vi "04 Loops.vi"() -> ()   [LabVIEW 2019]
uses:
  _Subs/OpenDiagram/Open_XControl.xctl
panel:
  in  "OpenDiag":refnum<vi>(xcontrol)
  out "Waveform Chart 3":i32[][](graph)
  out "Waveform Chart 2":i32(graph)
  out "Waveform Chart":i32(graph)
  # "04 Loops\nThis code compares while and for loops\n\nInstructions:\n1. Hit the Run arrow and see the plots change\n2. Look at the block diagram in Highlight Execution mode to see how data is fed to each chart"
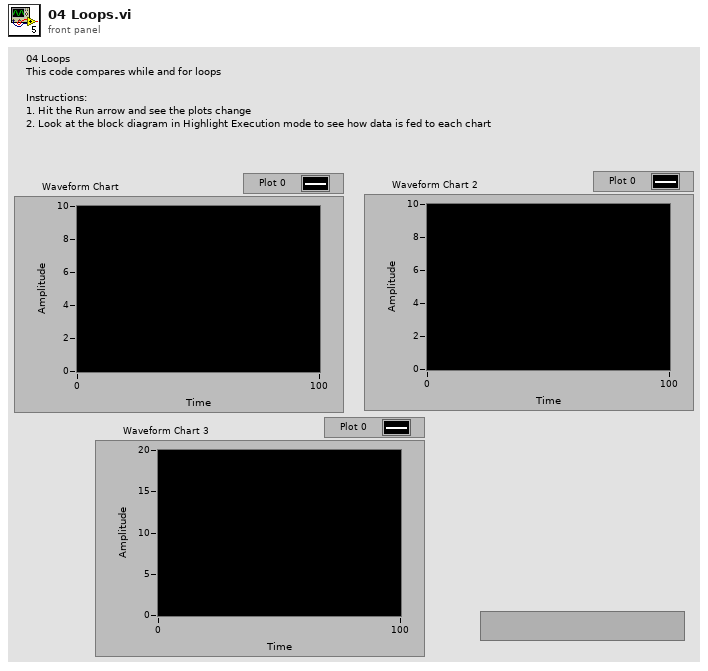
[diagram p1: front panel]
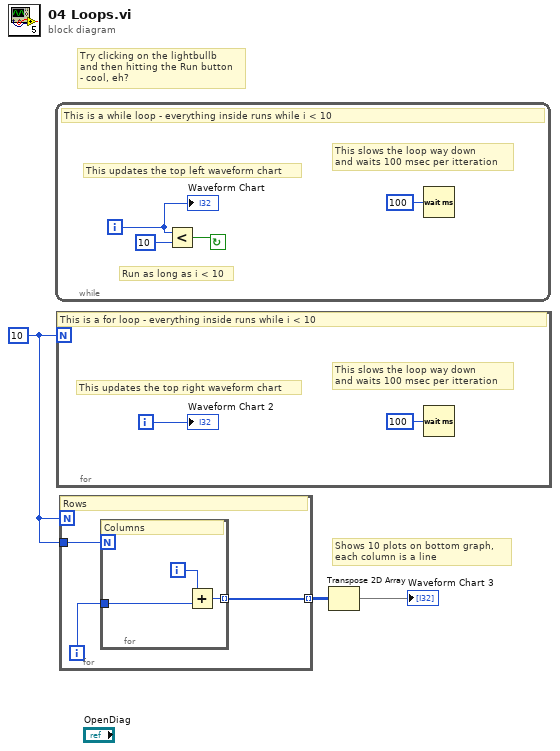
[diagram p0: block diagram]
diagram:
  w2 = 10
  # "Shows 10 plots on bottom graph,\neach column is a line"
  # "Try clicking on the lightbullb\nand then hitting the Run button\n- cool, eh?"
  n1 = while {
    i -> [w6]
    stop <- w4 continue-if-true
    # "Run as long as i < 10"
    # "This slows the loop way down \nand waits 100 msec per itteration"
    # "This updates the top left waveform chart"
    # "This is a while loop - everything inside runs while i < 10"
    n2 = Less?(x=w6, y=10) -> (x < y?=w4:bool)
    n3 = Wait (ms)(milliseconds to wait=u32 100) -> ()  [unwired: 1 out]
    "Waveform Chart" <- w6
  }
  n4 = for {
    N: w2 -> [_]
    i -> [w8]
    # "This slows the loop way down \nand waits 100 msec per itteration"
    # "This updates the top right waveform chart"
    # "This is a for loop - everything inside runs while i < 10"
    n5 = Wait (ms)(milliseconds to wait=u32 100) -> ()  [unwired: 1 out]
    "Waveform Chart 2" <- w8
  }
  n6 = for {
    N: w2 -> [_]
    tunnel: w2 -> [w12]
    tunnel: [w10] -> w3 mode=indexing
    i -> [w11]
    # "Rows"
    n7 = for {
      N: w12 -> [_]
      tunnel: w11 -> [w14]
      tunnel: [w13] -> w10 mode=indexing
      i -> [w15]
      # "Columns"
      n8 = Add(x=w15, y=w14) -> (x+y=w13:i32)
    }
  }
  n9 = Transpose 2D Array(2D array=w3) -> (transposed array=→"Waveform Chart 3":i32[][])
